vi "Get Total Physical Memory.vi"(8 "error in":errorcluster, 11 "Target IP Address":string) -> (0 "error out":errorcluster, 3 "Total Physical Memory (GB)":variant)   [LabVIEW 2026, in "Telemetry System Tests.lvclass"]
uses:
  Telemetry System Tests.lvclass
  <resource>/objmgr/nisysapi.rc
  <vilib>/nisyscfg/nisyscfg.lvlib
  <vilib>/nisyscfg/Close (System).vi
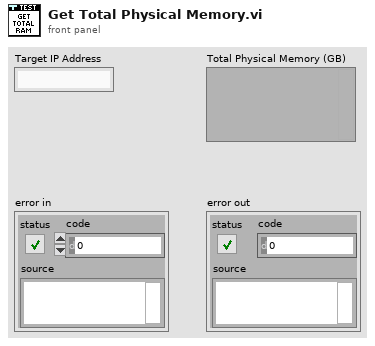
[diagram p1: front panel]
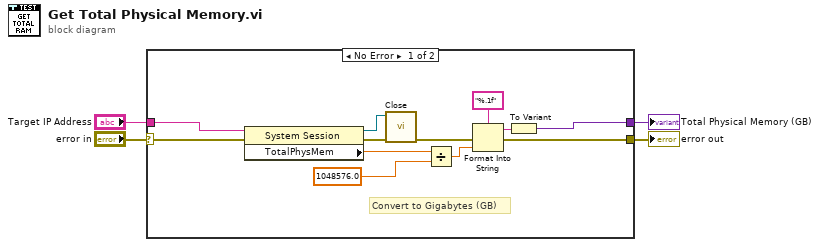
[diagram p0: block diagram]
diagram:
  n1 = case shown="No Error" "error in" {
    selector: "error in" -> [w9 w17]
    tunnel: [w16 _] -> w4
    tunnel: "Target IP Address" -> [w10 _]
    tunnel: [w5 w17] -> w2
    frame No Error {
      # "Convert to Gigabytes (GB)"
      n2 = property class="System Session"(reference=w10, error in=w9) -> (reference out=w6:refnum<k21>, error out=w8:errorcluster, "TotalPhysMem"=w11:dbl)
      n3 = call-poly <vilib>:"Close.vi"("error in (no error)"=w8, "Session in"=w6) -> ("error out"=w7:errorcluster)  [unwired: 9 in]
      n4 = Divide(x=w11, y=1048576.0) -> (x/y=w14:dbl)
      n5 = Format Into String(format string="%.1f", error in=w7, w14) -> (resulting string=w15:string, error out=w5:errorcluster)  [unwired: 1 in]
      n6 = To Variant(anything=w15) -> (Variant=w16:variant)
    }
    frame Error {
    }
  }
  "Total Physical Memory (GB)" <- w4
  "error out" <- w2
